vi "FM Radio.vi"() -> ()   [LabVIEW 2017]
uses:
  <vilib>/sound2/lvsound2.llb/Sound Data Format.ctl
  <vilib>/Analysis/baseanly.llb/Scale 1D.vi
  <vilib>/sound2/lvsound2.llb/Sound Output Set Volume (Single).vi
  <instrlib>/niUSRP/niUSRP Fetch Rx Data (CDB).vi
  <vilib>/Analysis/2dsp.llb/Resample (constant to constant,single -channel).vi
  <vilib>/sound2/lvsound2.llb/Sound Output Write (DBL).vi
  <vilib>/Analysis/NI_AALPro.lvlib
  <vilib>/ptbypt/NI_PtbyPt.lvlib
  <vilib>/Analysis/NI_AALBase.lvlib
panel:
  in  "A":dbl=10.0 format="%#_13g"
  in  "Configuration:Bandwidth":dbl=80000.0 format="%#_13p"
  in  "g2":dbl=0.00539258 format="%#_13g"
  in  "g1":dbl=0.10557 format="%#_13g"
  in  "method":T1(ring)
  in  "sound format 2":T2={"sample rate (S/s)"=44100.0, "number of channels"=1, "bits per sample"=32}
  in  "f_d":dbl=1000000.0 format="%#_13g"
  in  "gain 2":dbl=60.0 format="%#_6f"
  in  "device name 2":refnum<k15>="MyB210"
  in  "freq. 2":dbl=103900000.0 format="%#_6p"
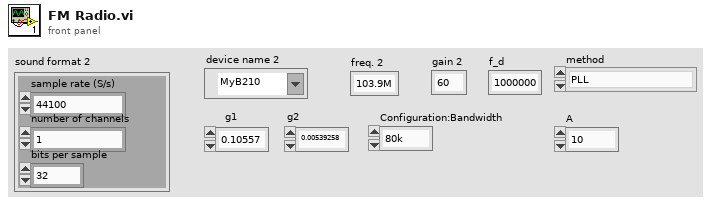
[diagram p1: front panel]
types:
  T1 = enum16{"PLL", "PPL without atan2", "differentiator", "differentiator unwrap", "differentiator conj"}
  T2 = typedef "Sound Data Format.ctl" = cluster{"sample rate (S/s)":dbl, "number of channels":i32, "bits per sample":i32}
  T3 = typedef "Sound Output Task ID.ctl" = u32
  T4 = cluster{"alias rejection (dB)":dbl, "normalized bandwidth":dbl}
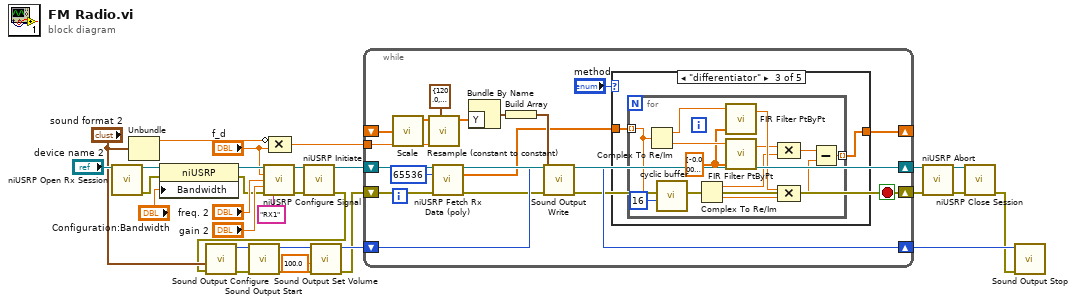
[diagram p0: block diagram]
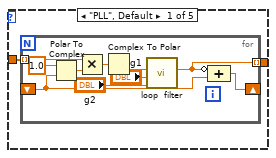
[diagram p2: hidden frame]
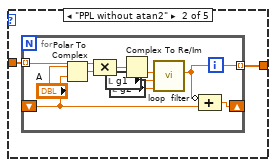
[diagram p3: hidden frame]
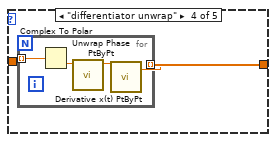
[diagram p4: hidden frame]
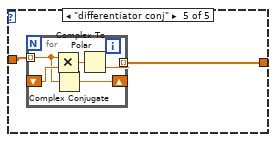
[diagram p5: hidden frame]
diagram:
  n1 = call <instrlib>:"niUSRP Open Rx Session.vi"("device names"="device name 2") -> ("session handle out"=w11:refnum<k15>, "error out"=w2:errorcluster)  [unwired: 13 in]
  n2 = Unbundle("sound format 2") -> ("sample rate (S/s)"=w4:dbl)  [unwired: 2 out]
  n3 = property class="niUSRP"(reference=w11, error in=w2, "Bandwidth"="Configuration:Bandwidth") -> (reference out=w10:refnum<k15>, error out=w1:errorcluster)
  n4 = call <instrlib>:"niUSRP Configure Signal.vi"("session handle"=w10, "IQ rate"="f_d", "carrier frequency"="freq. 2", "gain"="gain 2", "error in (no error)"=w1, "active antenna"="RX1") -> ("session handle out"=w26:refnum<k15>, "error out"=w25:errorcluster)  [unwired: 5 in, 3 out]
  n5 = Compound Arithmetic op=MULTIPLY(invert w4, "f_d") -> (w5:dbl)
  n6 = call <instrlib>:"niUSRP Initiate.vi"("session handle"=w26, "error in (no error)"=w25) -> ("session handle out"=w24:refnum<k15>, "error out"=w7:errorcluster)  [unwired: 12 in]
  n7 = call <vilib>:"Sound Output Configure.vi"("error in (no error)"=w7, "sound format"="sound format 2") -> ("error out"=w19:errorcluster, "task ID"=w18:T3)  [unwired: 8 in]
  n8 = call <vilib>:"Sound Output Start.vi"("error in (no error)"=w19, "task ID"=w18) -> ("error out"=w15:errorcluster, "task ID out"=w17:T3)  [unwired: 8 in]
  n9 = call-poly <vilib>:"Sound Output Set Volume.vi"("error in (no error)"=w15, "volume"=100.0, "task ID"=w17) -> ("error out"=w6:errorcluster, "task ID out"=w14:T3)  [unwired: 7 in]
  n10 = while {
    shift-right: [w38] -> w22
    shift-left: w6 -> [w48]
    shift-right: [w46] -> w20
    shift-left: w24 -> [w47]
    shift-right: [w43] -> w13
    shift-left: w14 -> [w44]
    shift-right: [w35] -> _
    shift-left: _ -> [w33]
    tunnel: w5 -> [w36]
    stop <- w38 stop-if-true
    n11 = call-poly <vilib>:"Scale.vi"("X"=w33) -> ("Y=(X-offset)/scale"=w32:dbl[])  [unwired: 3 out]
    n12 = call-poly <vilib>:"Resample (constant to constant).vi"("FIR filter specifications"=T4 {"alias rejection (dB)"=120.0, "normalized bandwidth"=0.25}, "dt"=w36, "X"=w32) -> ("Y"=w34:dbl[])  [unwired: 6 in, 2 out]
    n13 = call-poly <instrlib>:"niUSRP Fetch Rx Data (poly).vi"("session handle"=w47, "number of samples"=65536 ("channel 2"), "error in (no error)"=w48) -> ("session handle out"=w46:refnum<k15>, "data"=w31:cdb[], "error out"=w39:errorcluster)  [unwired: 9 in, 1 out]
    n14 = Bundle By Name("Y"=w34) -> (w42:waveform(dbl))  [unwired: 1 in]
    n15 = Build Array(w42) -> (w41:waveform(dbl)[])
    n16 = call-poly <vilib>:"Sound Output Write.vi"("error in (no error)"=w39, "data"=w41, "task ID"=w44) -> ("error out"=w38:errorcluster, "task ID out"=w43:T3)  [unwired: 7 in]
    n17 = case shown="\"differentiator\"" "method" {
      tunnel: w31 -> [w50 w61 w74 w89 w95]
      tunnel: [w49 w62 w73 w88 w94] -> w35
      frame "PLL", Default {
        n18 = for {
          tunnel: [w59] -> w49 mode=indexing
          tunnel: w50 -> [w51] mode=indexing
          shift-right: [w56] -> _
          shift-left: _ -> [w55]
          n19 = Polar To Complex(1:w55, 2:1.0 ("r")) -> (0:w52:cdb)
          n20 = Multiply(x=w51, y=w52) -> (x*y=w58:cdb)
          n21 = Complex To Polar(r * e^(i*theta)=w58) -> (theta=w57:dbl)  [unwired: 1 out]
          n22 = call "loop  filter.vi"("g2"="g2", "g1"="g1", "in"=w57) -> ("out"=w59:dbl)  [unwired: 8 in]
          n23 = Compound Arithmetic op=ADD(invert w59, w55) -> (w56:dbl)
        }
      }
      frame "PPL without atan2" {
        n24 = for {
          tunnel: [w66] -> w62 mode=indexing
          shift-right: [w69] -> _
          shift-left: _ -> [w68]
          tunnel: w61 -> [w65] mode=indexing
          n25 = Polar To Complex(1:w68, 2:"A") -> (0:w70:cdb)
          n26 = Compound Arithmetic op=MULTIPLY(w65, w70) -> (w72:cdb)
          n27 = local read "g1"() -> (w64:dbl)
          n28 = local read "g2"() -> (w63:dbl)
          n29 = Complex To Re/Im(x + iy=w72) -> (y=w67:dbl)  [unwired: 1 out]
          n30 = call "loop  filter.vi"("g2"=w63, "g1"=w64, "in"=w67) -> ("out"=w66:dbl)  [unwired: 8 in]
          n31 = Compound Arithmetic op=ADD(invert w66, w68) -> (w69:dbl)
        }
      }
      frame "differentiator" {
        n32 = for {
          tunnel: w74 -> [w79] mode=indexing
          tunnel: [w80] -> w73 mode=indexing
          w81 = dbl[] [-0.000659109772935775, 0.0014309460615869565, -0.001899623787887634, 0.0027365129408949635, -0.003835594807064277, 0.005232625488704574, -0.006988406311111355, 0.009186676314476925, -0.01195054040147665, 0.015467596710993431, -0.020047742424394645, 0.026250702416797195, -0.035201300639023506, 0.04953741985580705, -0.07719915466301731, 0.15795504262477333, 0.0, -0.15795504262477333, 0.07719915466301731, -0.04953741985580705, 0.035201300639023506, -0.026250702416797195, 0.020047742424394645, -0.015467596710993431, 0.01195054040147665, -0.009186676314476925, 0.006988406311111355, -0.005232625488704574, 0.003835594807064277, -0.0027365129408949635, 0.001899623787887634, -0.0014309460615869565, 0.000659109772935775] ("110,25k     33taps")
          n33 = Complex To Re/Im(x + iy=w79) -> (x=w84:dbl, y=w83:dbl)
          n34 = call "cyclic buffer.vi"("dimension size"=16 ("sample length"), "new element"=w79) -> ("delayed \nelement"=w78:cdb)  [unwired: 9 in]
          n35 = Complex To Re/Im(x + iy=w78) -> (x=w75:dbl, y=w77:dbl)
          n36 = call <vilib>:"FIR Filter PtByPt.vi"("Forward Coefficients"=w81, "x"=w84) -> ("Filtered x"=w87:dbl)  [unwired: 2 in, 1 out]
          n37 = call <vilib>:"FIR Filter PtByPt.vi"("Forward Coefficients"=w81, "x"=w83) -> ("Filtered x"=w76:dbl)  [unwired: 2 in, 1 out]
          n38 = Compound Arithmetic op=MULTIPLY(w76, w75) -> (w86:dbl)
          n39 = Compound Arithmetic op=MULTIPLY(w87, w77) -> (w85:dbl)
          n40 = Subtract(x=w86, y=w85) -> (x-y=w80:dbl)
        }
      }
      frame "differentiator unwrap" {
        n41 = for {
          tunnel: w89 -> [w91] mode=indexing
          tunnel: [w90] -> w88 mode=indexing
          n42 = Complex To Polar(r * e^(i*theta)=w91) -> (theta=w93:dbl)  [unwired: 1 out]
          n43 = call <vilib>:"Unwrap Phase PtByPt.vi"("phase"=w93) -> ("unwrapped phase"=w92:dbl)  [unwired: 10 in]
          n44 = call <vilib>:"Derivative x(t) PtByPt.vi"("x"=w92) -> ("dx/dt"=w90:dbl)  [unwired: 3 in, 1 out]
        }
      }
      frame "differentiator conj" {
        n45 = for {
          tunnel: [w96] -> w94 mode=indexing
          tunnel: w95 -> [w98] mode=indexing
          shift-right: [w97] -> _
          shift-left: _ -> [w99]
          n46 = Multiply(x=w98, y=w99) -> (x*y=w100:cdb)
          n47 = Complex Conjugate(1:w98) -> (0:w97:cdb)
          n48 = Complex To Polar(r * e^(i*theta)=w100) -> (theta=w96:dbl)  [unwired: 1 out]
        }
      }
    }
  }
  n49 = call <instrlib>:"niUSRP Abort.vi"("session handle"=w20, "error in (no error)"=w22) -> ("session handle out"=w23:refnum<k15>, "error out"=w21:errorcluster)  [unwired: 12 in]
  n50 = call <instrlib>:"niUSRP Close Session.vi"("session handle"=w23, "error in (no error)"=w21) -> ("error out"=w8:errorcluster)  [unwired: 13 in]
  n51 = call <vilib>:"Sound Output Stop.vi"("error in (no error)"=w8, "task ID"=w13) -> ()  [unwired: 8 in, 2 out]
